vi "t03_2020.vi"() -> ()   [LabVIEW 2021]
uses:
  <vilib>/Utility/file.llb/Write Delimited Spreadsheet (string).vi
panel:
  out "array":string[](array[string])
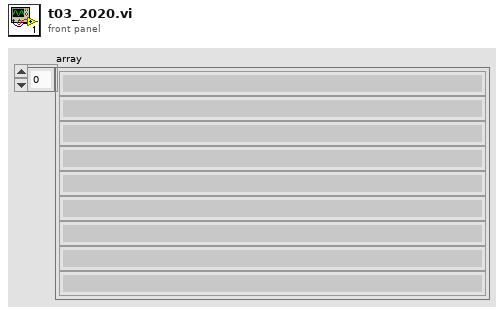
[diagram p1: front panel]
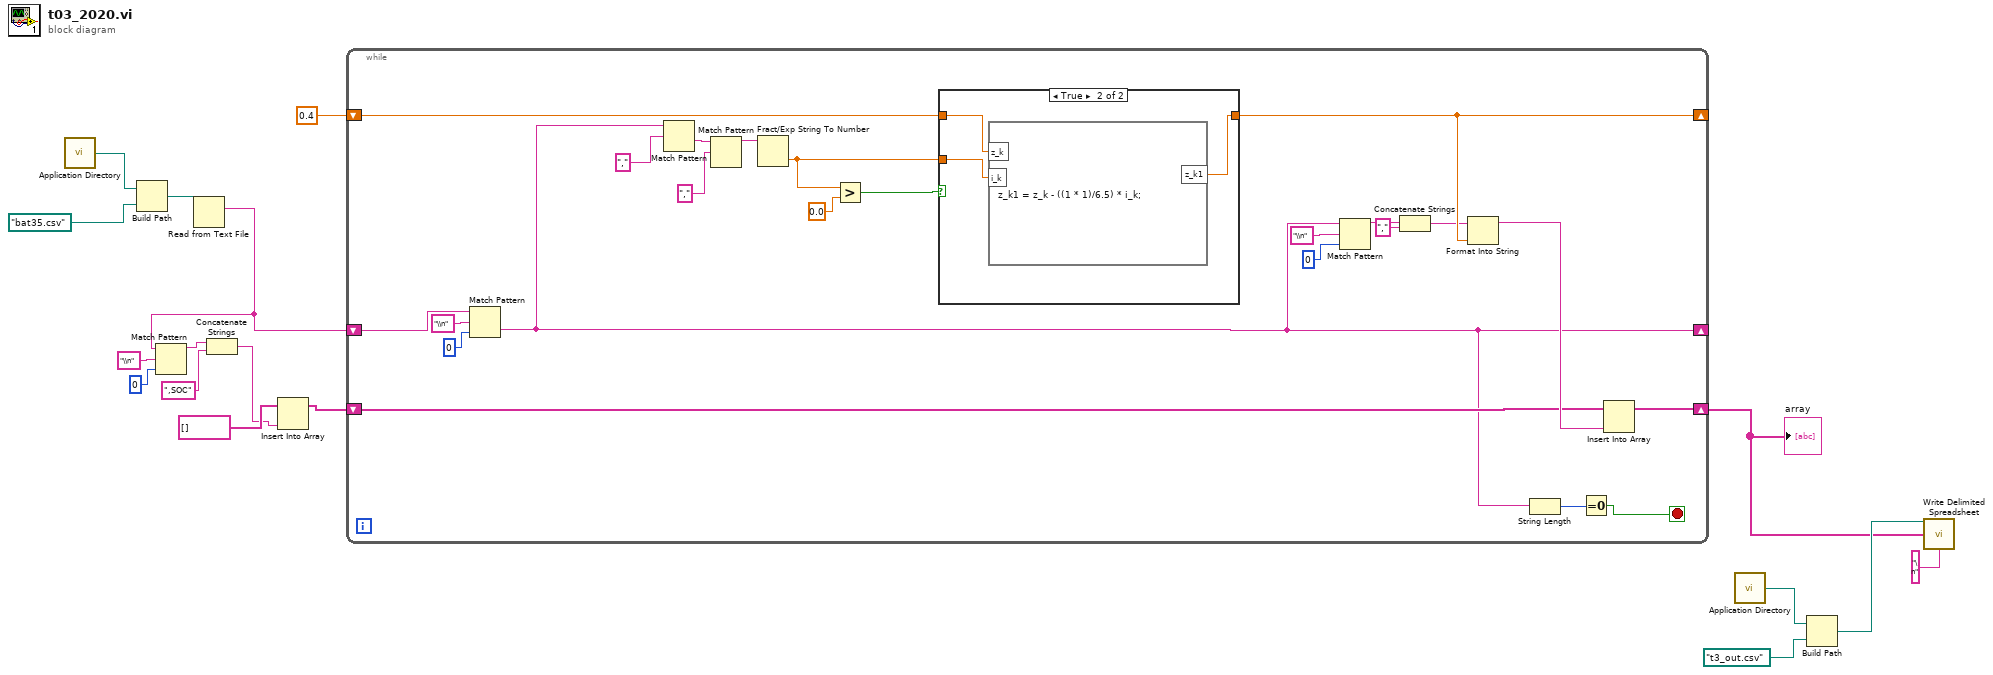
[diagram p0: block diagram]
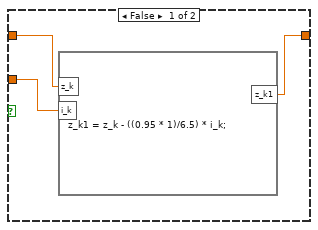
[diagram p2: hidden frame]
diagram:
  n1 = call <vilib>:"Application Directory.vi"() -> ("Application Directory"=w17:path)
  n2 = Build Path(base path=w17, name or relative path=path "bat35.csv" ("file (use dialog)")) -> (appended path=w15:path)
  n3 = Read from Text File(file (use dialog)=w15) -> (text=w11:string)  [unwired: 3 in, 3 out]
  n4 = Match Pattern(string=w11, regular expression="\\n", offset (0)=0) -> (before substring=w8:string)  [unwired: 3 out]
  n5 = Concatenate Strings(w8, ",SOC" ("string")) -> (w7:string)
  n6 = Insert Into Array "Insert Into Array"(array=string[] [], new element=w7) -> (w9:string[])  [unwired: 1 in]
  n7 = while {
    shift-right: [w18] -> _
    shift-left: w11 -> [w40]
    shift-right: [w27] -> _
    shift-left: 0.4 -> [w31]
    shift-right: [w23] -> w1
    shift-left: w9 -> [w20]
    stop <- w19 stop-if-true
    n8 = Match Pattern(string=w40, regular expression="\\n", offset (0)=0) -> (after substring=w18:string)  [unwired: 3 out]
    n9 = Match Pattern(string=w18, regular expression=",") -> (after substring=w34:string)  [unwired: 1 in, 3 out]
    n10 = Match Pattern(string=w34, regular expression=",") -> (before substring=w35:string)  [unwired: 1 in, 3 out]
    n11 = Fract/Exp String To Number(string=w35) -> (number=w30:dbl)  [unwired: 3 in, 1 out]
    n12 = Greater?(x=w30, y=0.0) -> (0:w32:bool)
    n13 = case shown="True" w32 {
      tunnel: w31 -> [w43 w46]
      tunnel: [w41 w45] -> w27
      tunnel: w30 -> [w42 w44]
      frame False {
        n14 = formula code="z_k1 = z_k - ((0.95 * 1)/6.5) * i_k;"("z_k"=w43, "i_k"=w42) -> ("z_k1"=w41:dbl)
      }
      frame True {
        n15 = formula code="z_k1 = z_k - ((1 * 1)/6.5) * i_k;"("z_k"=w46, "i_k"=w44) -> ("z_k1"=w45:dbl)
      }
    }
    n16 = Match Pattern(string=w18, regular expression="\\n", offset (0)=0) -> (before substring=w26:string)  [unwired: 3 out]
    n17 = Concatenate Strings(w26, "," ("string")) -> (w24:string)
    n18 = Format Into String(initial string=w24, w27) -> (resulting string=w22:string)  [unwired: 2 in, 1 out]
    n19 = String Length(string=w18) -> (length=w21:i32)
    n20 = Equal To 0?(x=w21) -> (x = 0?=w19:bool)
    n21 = Insert Into Array "Insert Into Array"(array=w20, new element=w22) -> (w23:string[])  [unwired: 1 in]
  }
  "array" <- w1
  n22 = call <vilib>:"Application Directory.vi"() -> ("Application Directory"=w5:path)
  n23 = Build Path(base path=w5, name or relative path=path "t3_out.csv" ("file (use dialog)")) -> (appended path=w3:path)
  n24 = call-poly <vilib>:"Write Delimited Spreadsheet.vi"("file path (dialog if empty)"=w3, "1D data"=w1, "delimiter (\\t)"="\n" ("delimiter (\\t)")) -> ()  [unwired: 11 in, 2 out]
